vi "WebDAV mass transfer.vi"(11 "Prevented Files":path[](array[path])) -> ()   [LabVIEW 2019]
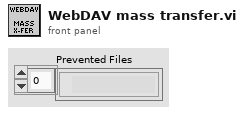
[diagram p1: front panel]
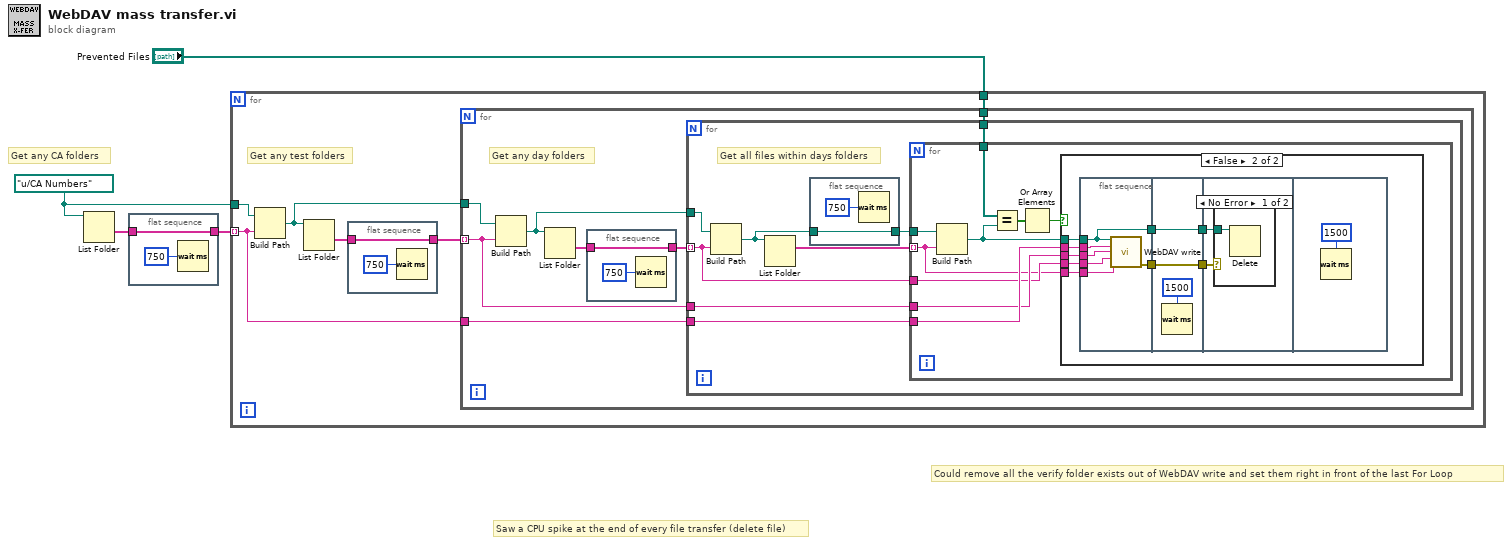
[diagram p0: block diagram]
diagram:
  w4 = path "u:/CA Numbers"
  # "Could remove all the verify folder exists out of WebDAV write and set them right in front of the last For Loop"
  # "Saw a CPU spike at the end of every file transfer (delete file)"
  # "Get any CA folders"
  n1 = List Folder(path=w4) -> (folder names=w2:string[])  [unwired: 3 in, 3 out]
  n2 = flat-sequence {
    tunnel: w2 -> [w5]
    tunnel: [w5] -> w1
    frame #0 {
      n3 = Wait (ms)(milliseconds to wait=u32 750) -> ()  [unwired: 1 out]
    }
  }
  n4 = for {
    tunnel: w1 -> [w9] mode=indexing
    tunnel: w4 -> [w12]
    tunnel: "Prevented Files" -> [w10]
    # "Get any test folders"
    n5 = Build Path(base path=w12, name or relative path=w9) -> (appended path=w11:path)
    n6 = List Folder(path=w11) -> (folder names=w8:string[])  [unwired: 3 in, 3 out]
    n7 = flat-sequence {
      tunnel: w8 -> [w13]
      tunnel: [w13] -> w7
      frame #0 {
        n8 = Wait (ms)(milliseconds to wait=u32 750) -> ()  [unwired: 1 out]
      }
    }
    n9 = for {
      tunnel: w11 -> [w20]
      tunnel: w7 -> [w17] mode=indexing
      tunnel: w10 -> [w21]
      tunnel: w9 -> [w18]
      # "Get any day folders"
      n10 = Build Path(base path=w20, name or relative path=w17) -> (appended path=w19:path)
      n11 = List Folder(path=w19) -> (folder names=w16:string[])  [unwired: 3 in, 3 out]
      n12 = flat-sequence {
        tunnel: w16 -> [w22]
        tunnel: [w22] -> w15
        frame #0 {
          n13 = Wait (ms)(milliseconds to wait=u32 750) -> ()  [unwired: 1 out]
        }
      }
      n14 = for {
        tunnel: w15 -> [w29] mode=indexing
        tunnel: w19 -> [w31]
        tunnel: w21 -> [w28]
        tunnel: w18 -> [w27]
        tunnel: w17 -> [w26]
        # "Get all files within days folders"
        n15 = Build Path(base path=w31, name or relative path=w29) -> (appended path=w25:path)
        n16 = List Folder(path=w25) -> (filenames=w30:string[])  [unwired: 3 in, 3 out]
        n17 = flat-sequence {
          tunnel: w25 -> [w32]
          tunnel: [w32] -> w24
          frame #0 {
            n18 = Wait (ms)(milliseconds to wait=u32 750) -> ()  [unwired: 1 out]
          }
        }
        n19 = for {
          tunnel: w30 -> [w34] mode=indexing
          tunnel: w24 -> [w42]
          tunnel: w29 -> [w35]
          tunnel: w28 -> [w41]
          tunnel: w27 -> [w37]
          tunnel: w26 -> [w36]
          n20 = Build Path(base path=w42, name or relative path=w34) -> (appended path=w40:path)
          n21 = Equal?(x=w41, y=w40) -> (x = y?=w39:bool[])
          n22 = Or Array Elements(Boolean array=w39) -> (logical OR=w38:bool)
          n23 = case shown="False" w38 {
            tunnel: w37 -> [_ w51]
            tunnel: w35 -> [_ w50]
            tunnel: w36 -> [_ w49]
            tunnel: w40 -> [_ w48]
            tunnel: w34 -> [_ w47]
            frame True {
              # "Don't transfer either\nof the current files"
            }
            frame False {
              n24 = flat-sequence {
                tunnel: w48 -> [w52]
                tunnel: w51 -> [w57]
                tunnel: w50 -> [w55]
                tunnel: w49 -> [w56]
                tunnel: w47 -> [w54]
                tunnel: [w53] -> w46
                tunnel: [w52] -> w43
                tunnel: w46 -> [w59]
                tunnel: [w59] -> w45
                tunnel: [w58] -> w44
                tunnel: w43 -> [w58]
                tunnel: w45 -> [w62]
                tunnel: w44 -> [w61]
                frame #0 {
                  n25 = call "WebDAV write.vi"("RIO Filepath"=w52, "CA Number"=w57, "Test Name"=w56, "Date"=w55, "Filename"=w54) -> ("error out"=w53:errorcluster)  [unwired: 10 in]
                }
                frame #1 {
                  n26 = Wait (ms)(milliseconds to wait=u32 1500) -> ()  [unwired: 1 out]
                }
                frame #2 {
                  n27 = case shown="No Error" w62 {
                    tunnel: w61 -> [w63 _]
                    frame No Error {
                      n28 = Delete(path (use dialog)=w63) -> ()  [unwired: 4 in, 3 out]
                    }
                    frame Error {
                    }
                  }
                }
                frame #3 {
                  n29 = Wait (ms)(milliseconds to wait=u32 1500) -> ()  [unwired: 1 out]
                }
              }
            }
          }
        }
      }
    }
  }
